vi "Test Line Intersection.vi"(11 "Test Case In":refnum<class "Collision Tests.lvclass">) -> (0 "error out":errorcluster, 3 "Test Case Out":refnum<class "Collision Tests.lvclass">)   [LabVIEW 2021, in "Collision Tests.lvclass"]
uses:
  Collision Tests.lvclass
  Re-use Libraries/Collision/Collision.lvlib
  Re-use Libraries/Vector 2D/Vector 2D.lvclass
  Re-use Libraries/Utility/Utility.lvlib
  <vilib>/picture/picture.llb/Draw True-Color Pixmap.vi
panel:
  out "new picture":picture
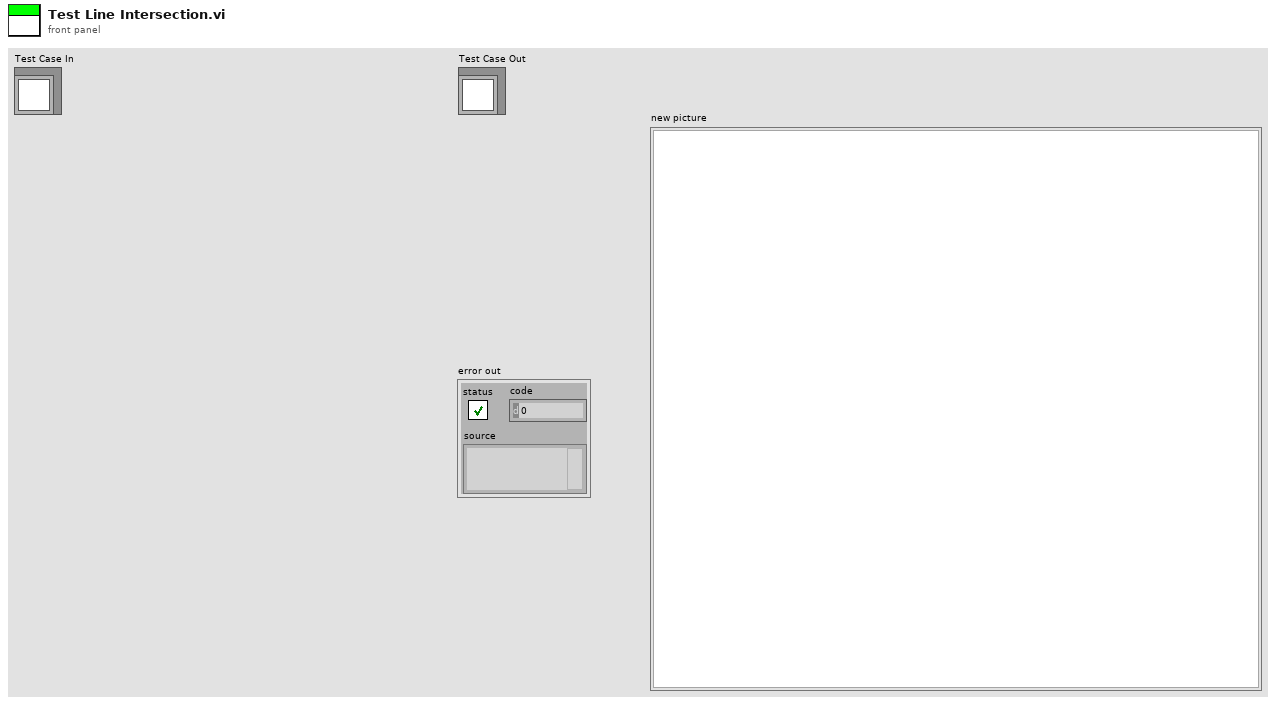
[diagram p1: front panel]
types:
  T1 = cluster{"left":i16, "top":i16, "right":i16, "bottom":i16}
  T2 = typedef "imagedata.ctl" = cluster{"image type":i32, "image depth":i32, "image":u8[], "mask":u8[], "colors":u32[], "Rectangle":cluster{"left":i16, "top":i16, "right":i16, "bottom":i16}}
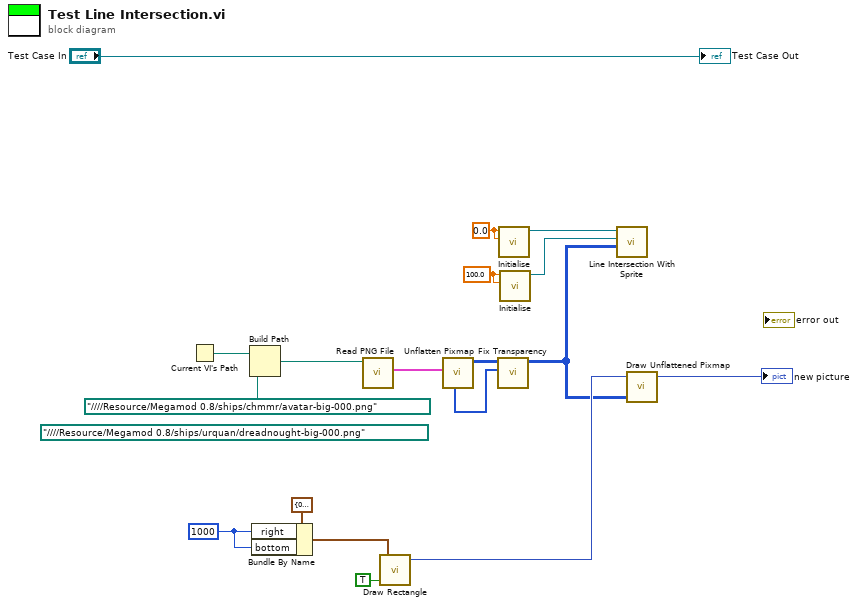
[diagram p0: block diagram]
diagram:
  (unwired) path "../../../../Resource/Megamod 0.8/ships/urquan/dreadnought-big-000.png" ("Path")
  w8 = i16 1000 ("right")
  w15 = sgl 100.0 ("x")
  w16 = sgl 0.0 ("x")
  n1 = Current VI's Path() -> (path=w14:path)
  n2 = Build Path(base path=w14, name or relative path=path "../../../../Resource/Megamod 0.8/ships/chmmr/avatar-big-000.png" ("Path")) -> (appended path=w12:path)
  n3 = Bundle By Name(cluster=T1 {"left"=0, "top"=0, "right"=0, "bottom"=0} ("rect"), "right"=w8, "bottom"=w8) -> (w10:T1)
  n4 = call <vilib>:"Read PNG File.vi"("path to PNG file"=w12) -> ("image data"=w7:T2)  [unwired: 8 in, 2 out]
  n5 = call <vilib>:"Draw Rectangle.vi"("rect"=w10, "fill?(F)"=TRUE) -> ("new picture"=w6:picture)  [unwired: 7 in]
  n6 = call <vilib>:"Unflatten Pixmap.vi"("image data"=w7) -> ("24-bit pixmap"=w3:u32[][], "mask"=w4:u8[])  [unwired: 4 in, 5 out]
  n7 = call "Fix Transparency.vi"("Mask"=w4, "Pixels In"=w3) -> ("Pixels Out"=w2:u32[][])  [unwired: 9 in]
  n8 = call "Initialise.vi"("y"=w16, "x"=w16) -> ("Vector 2D out"=w18:refnum<class "Vector 2D.lvclass">)  [unwired: 9 in]
  n9 = call "Initialise.vi"("y"=w15, "x"=w15) -> ("Vector 2D out"=w17:refnum<class "Vector 2D.lvclass">)  [unwired: 9 in]
  n10 = call "Line Intersection With Sprite.vi"("Pixel Data in"=w2, "Line End Point"=w17, "Line Start Point"=w18) -> ()  [unwired: 7 in, 2 out]
  n11 = call-poly <vilib>:"Draw Unflattened Pixmap.vi"("picture"=w6, "data (RGB format)"=w2) -> ("new picture"=→"new picture":picture)  [unwired: 7 in]
  "Test Case Out" <- "Test Case In"
